vi "探头窗口-6-服务器版.vi"() -> ()   [LabVIEW 2013]
panel:
  in  "外部停止命令？":bool=TRUE
  out "引用-探头属性[]":refnum<vi>
  out "引用-监测模式？":refnum<vi>
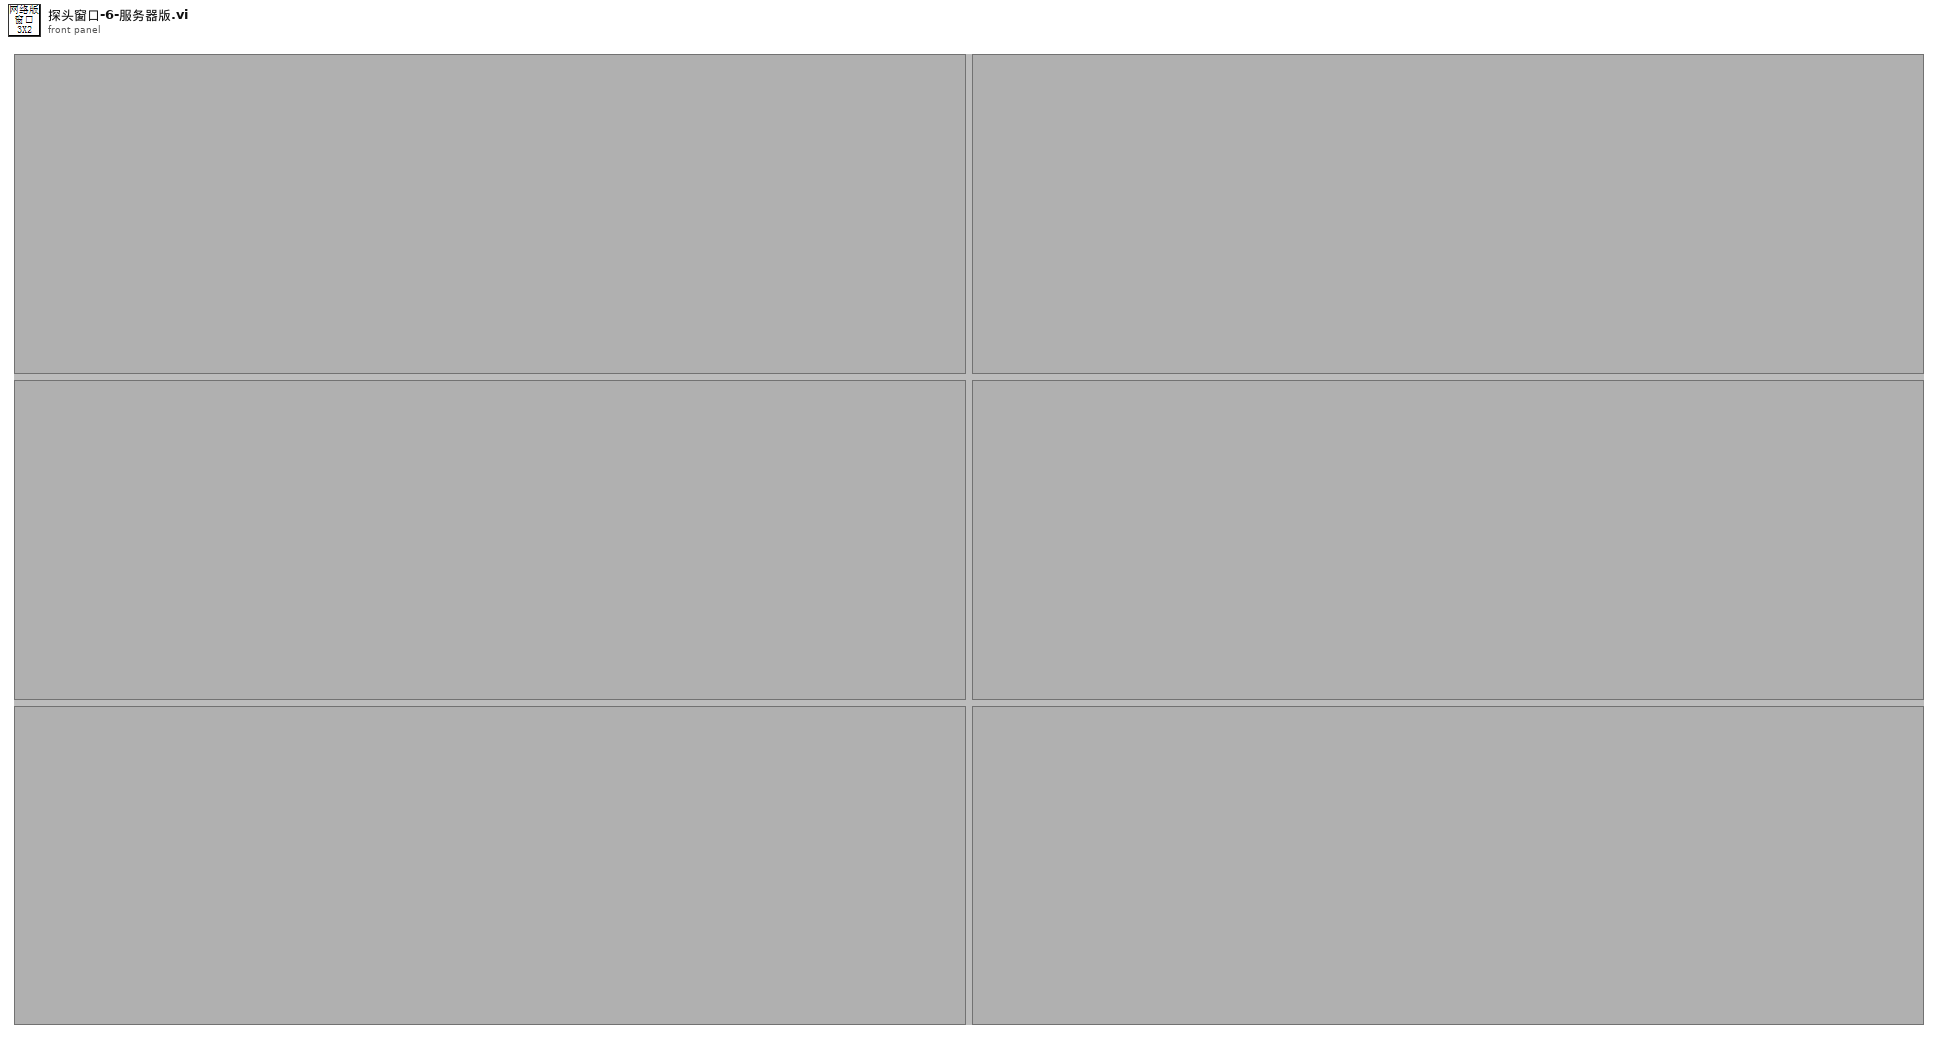
[diagram p1: front panel]
types:
  T1 = cluster{"探头地址与信息":cluster{"网络地址":cluster{"IP":string, "port":u16}, "探头信息":string}, "测量值":cluster{"时间":timestamp, "数值":dbl}, "限值":cluster{"限值1":dbl, "限值2":dbl}, "探头状态":enum16{"正常", "离线", "禁用", "一级报警", "二级报警"}}[]
  T2 = typedef "eventvkey.ctl" = enum16{"ASCII", "Enter", "Return", "Shift", "Ctrl", "Alt", "Cmd", "Opt", "Caps", "NumLock", "Clear", "Break", "Up", "Down", "Left", "Right", "Insert", "Delete", "Home", "End", "PageUp", "PageDown", "Escape", "Help", "Pause", "ScrollLock", "F1", "F2", "F3", "F4", "F5", "F6", "F7", "F8", "F9", "F10", "F11", "F12", "F13", "F14", "F15", "F16", "F17", "F18", "F19", "F20", "F21", "F22", "F23", "F24", "Play", "VolumeUp", "VolumeDown", "Mute", "Two Byte Char"}
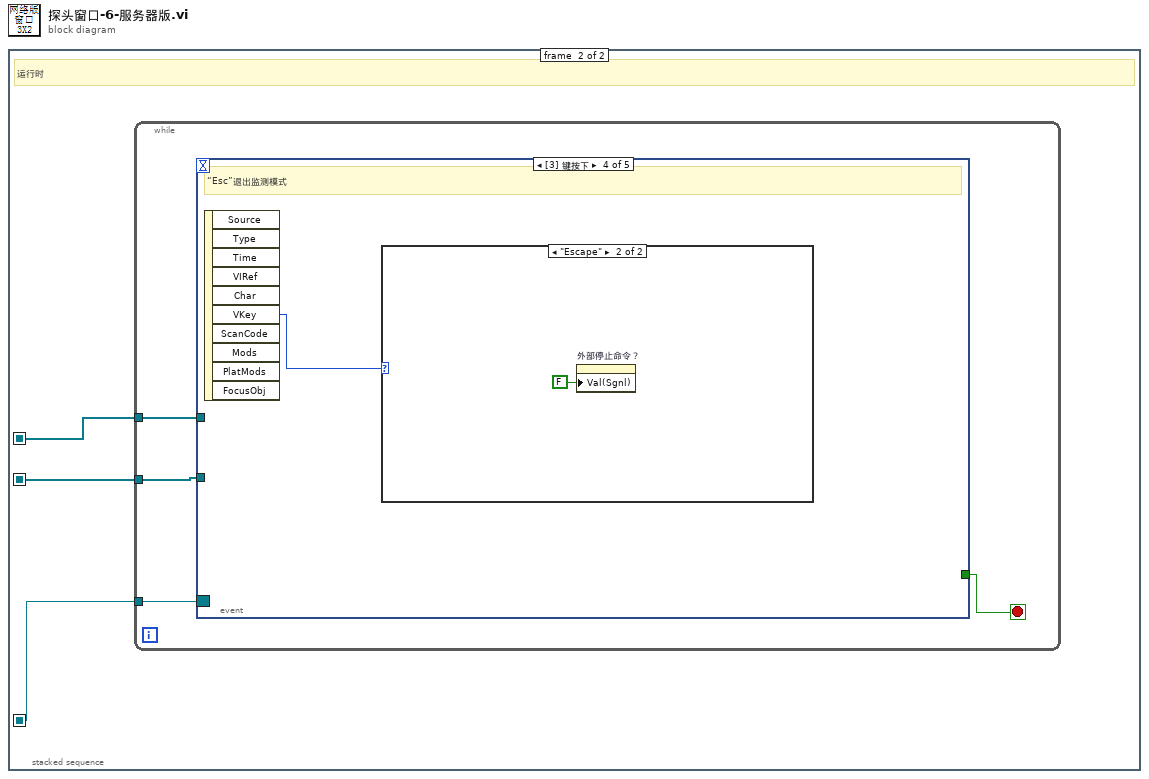
[diagram p0: block diagram]
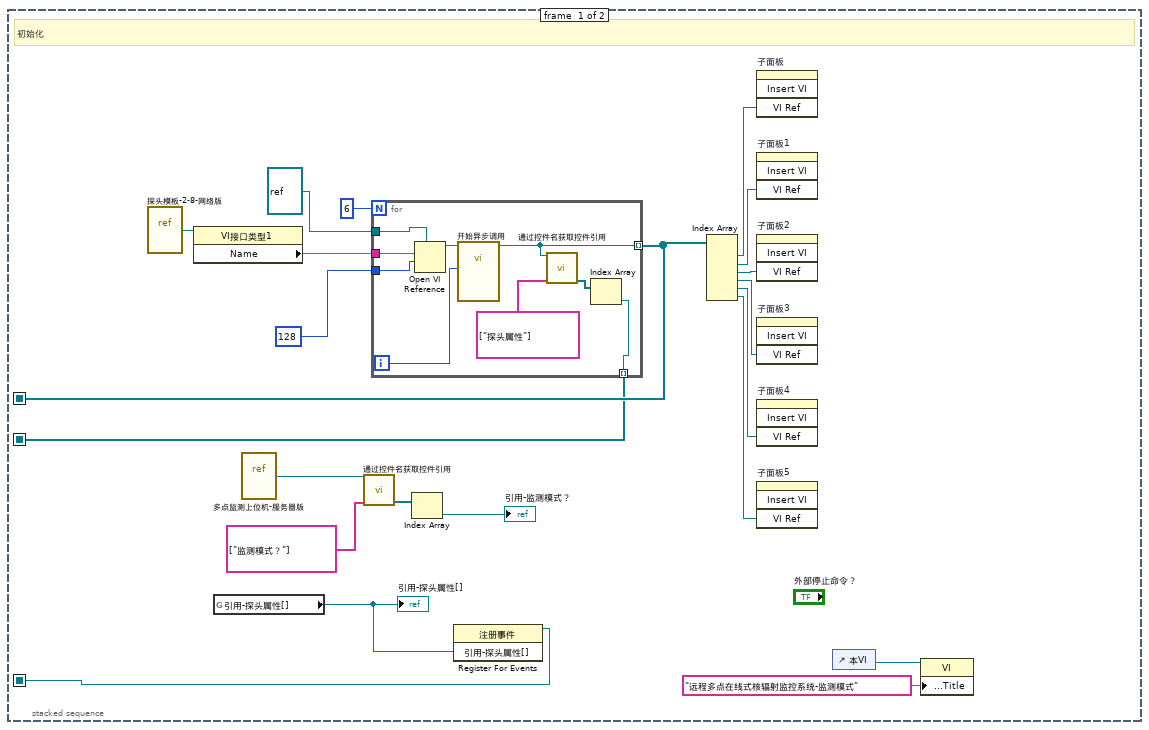
[diagram p2: hidden frame]
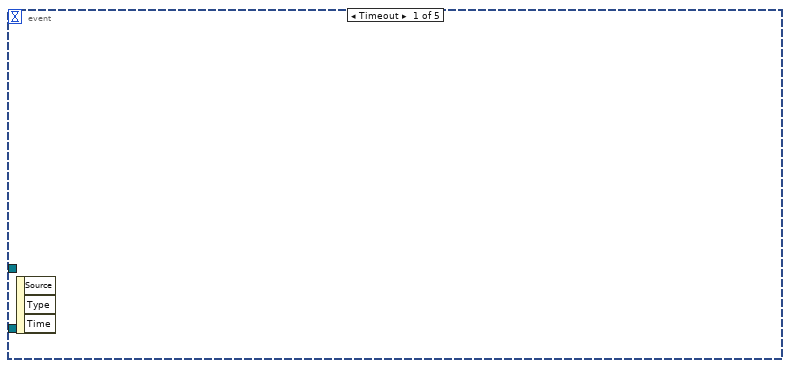
[diagram p3: hidden frame]
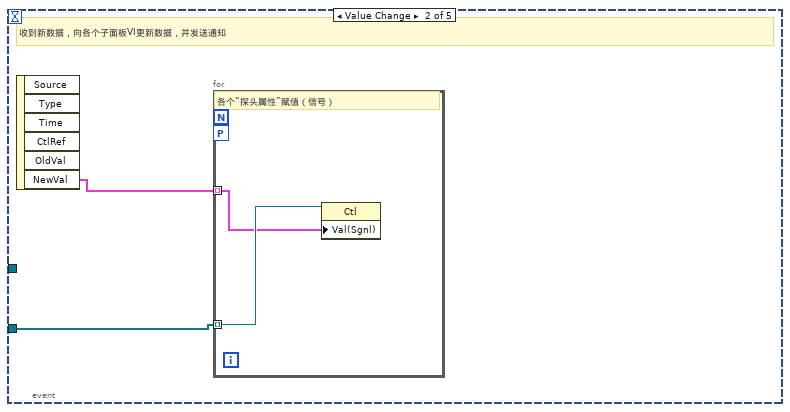
[diagram p4: hidden frame]
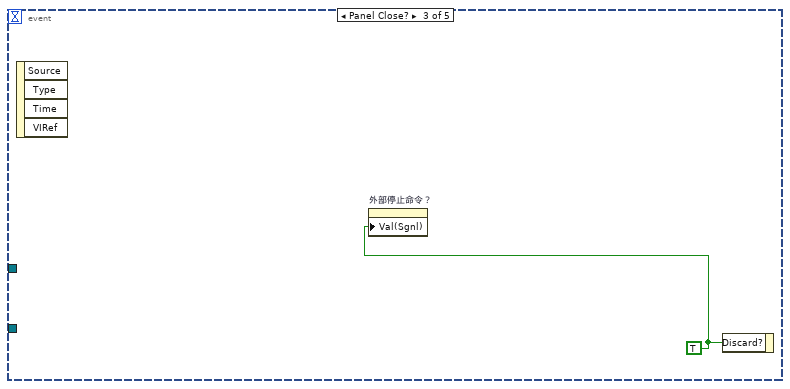
[diagram p5: hidden frame]
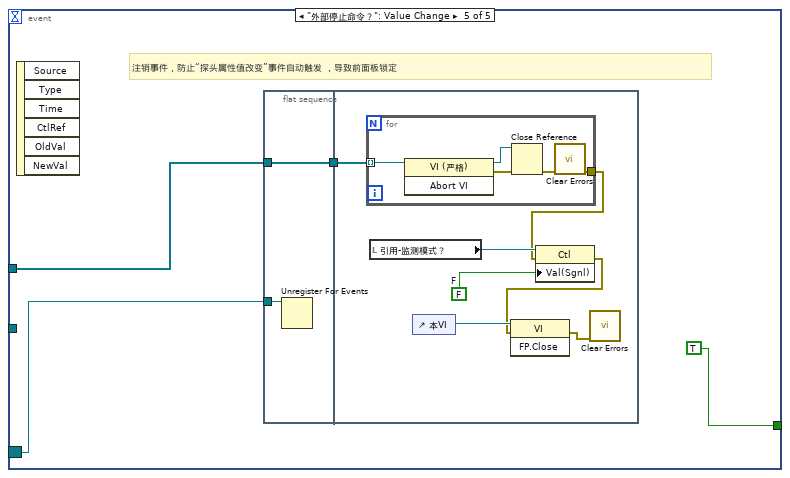
[diagram p7: hidden frame]
diagram:
  n1 = stacked-sequence {
    seq-local: [w17 _] -> [_ w33]
    seq-local: [w9 _] -> [_ w32]
    seq-local: [w3 _] -> [_ w31]
    frame #0 {
      # "初始化"
      n2 = vi-ref "探头模板-2-8-网络版.vi"() -> (w21:refnum<vi>)
      n3 = property class="VI接口类型1"(reference=w21) -> ("Name"=w20:string)  [unwired: 1 in, 2 out]
      n4 = global read "全局变量-35点监测.vi" "引用-探头属性[]"() -> (w4:refnum<vi>)
      "引用-探头属性[]" <- w4
      n5 = vi-ref "多点监测上位机-服务器版.vi"() -> (w5:refnum<vi>)
      n6 = call "通过控件名获取控件引用.vi"("控件名数组"=string[] ["监测模式？"], "VI引用"=w5) -> ("控件引用输出"=w7:refnum<vi>[])  [unwired: 7 in, 2 out]
      n7 = for {
        N: 6 -> [_]
        tunnel: w20 -> [w30]
        tunnel: 128 ("选项") -> [w29]
        tunnel: refnum<vi> refnum ("类型说明符VI引用句柄（仅用于类型）") -> [w28]
        tunnel: [w23] -> w17 mode=indexing
        tunnel: [w24] -> w9 mode=indexing
        i -> [w22]
        n8 = Open VI Reference(type specifier VI Refnum (for type only)=w28, vi path=w30, options=w29) -> (vi reference=w25:refnum<vi>)  [unwired: 3 in, 1 out]
        n9 = call-by-ref "开始异步调用"(reference=w25, "探头序号"=w22) -> (reference out=w23:refnum<vi>)  [unwired: 12 in, 1 out]
        n10 = call "通过控件名获取控件引用.vi"("控件名数组"=string[] ["探头属性"], "VI引用"=w23) -> ("控件引用输出"=w27:refnum<vi>[])  [unwired: 7 in, 2 out]
        n11 = Index Array(array=w27) -> (element=w24:refnum<vi>)  [unwired: 1 in]
      }
      n12 = Index Array(array=w7) -> (element=→"引用-监测模式？":refnum<vi>)  [unwired: 1 in]
      n13 = register-events(w4) -> (reference out=w3:refnum<event-registration>)  [unwired: 2 in, 1 out]
      n14 = Index Array(array=w17) -> (element #1=w15:refnum<vi>, element #2=w14:refnum<vi>, element #3=w13:refnum<vi>, element #4=w12:refnum<vi>, element #5=w10:refnum<vi>, element #6=w11:refnum<vi>)  [unwired: 6 in]
      n15 = invoke on="子面板" class="子面板" method="Insert VI"("VI Ref"=w15) -> ()  [unwired: 3 in, 4 out]
      n16 = invoke on="子面板1" class="SubPnl" method="Insert VI"("VI Ref"=w14) -> ()  [unwired: 3 in, 4 out]
      n17 = invoke on="子面板2" class="SubPnl" method="Insert VI"("VI Ref"=w13) -> ()  [unwired: 3 in, 4 out]
      n18 = invoke on="子面板3" class="SubPnl" method="Insert VI"("VI Ref"=w12) -> ()  [unwired: 3 in, 4 out]
      n19 = invoke on="子面板4" class="SubPnl" method="Insert VI"("VI Ref"=w10) -> ()  [unwired: 3 in, 4 out]
      n20 = invoke on="子面板5" class="SubPnl" method="Insert VI"("VI Ref"=w11) -> ()  [unwired: 3 in, 4 out]
      n21 = control-ref of="本VI"() -> (w2:refnum<vi>)
      n22 = property class="VI"(reference=w2, "Front Panel.Title"="远程多点在线式核辐射监控系统-监测模式" ("前面板窗口:标题")) -> ()  [unwired: 1 in, 2 out]
    }
    frame #1 {
      # "运行时"
      n23 = while {
        tunnel: w33 -> [w36]
        tunnel: w32 -> [w35]
        tunnel: w31 -> [w34]
        stop <- w37 stop-if-true
        n24 = event shown="[3] 键按下" {
          selector: w34 -> [_ _ _ _ w45]
          dyn-events: _ -> [_ _ _ _ _]
          timeout: _ -> [_ _ _ _ _]
          tunnel: [_ _ _ _ TRUE ("放弃？")] -> w37
          tunnel: w36 -> [_ _ _ _ w47]
          tunnel: w35 -> [_ w38 _ _ _]
          event Timeout {
            n25 = event-data() -> ()  [unwired: 1 in, 3 out]
          }
          event Value Change {
            # "收到新数据，向各个子面板VI更新数据，并发送通知"
            n26 = event-data() -> ("NewVal"=w39:T1)  [unwired: 1 in, 5 out]
            n27 = for {
              workers-P: _ -> [_]
              tunnel: w38 -> [w41] mode=indexing
              tunnel: w39 -> [w40] mode=indexing
              # "各个“探头属性”赋值（信号）"
              n28 = property class="Ctl"(reference=w41, "Val(Sgnl)"=w40) -> ()  [unwired: 1 in, 2 out]
            }
          }
          event Panel Close? {
            w42 = TRUE ("放弃？")
            n29 = event-data() -> ()  [unwired: 1 in, 4 out]
            n30 = property on="外部停止命令？" class="Bool (严格)"("Val(Sgnl)"=w42) -> ()  [unwired: 2 in, 2 out]
            n31 = event-data("Discard?"=w42) -> ()  [unwired: 1 in, 1 out]
          }
          event Key Down {
            # "“Esc”退出监测模式"
            n32 = event-data() -> ("VKey"=w43:T2)  [unwired: 1 in, 9 out]
            n33 = case shown="\"Escape\"" w43 {
              frame "ASCII", Default {
              }
              frame "Escape" {
                n34 = property on="外部停止命令？" class="Bool (严格)"("Val(Sgnl)"=FALSE ("值(信号)")) -> ()  [unwired: 2 in, 2 out]
              }
            }
          }
          event "外部停止命令？": Value Change {
            # "注销事件，防止“探头属性值改变”事件自动触发 ，导致前面板锁定"
            n35 = event-data() -> ()  [unwired: 1 in, 6 out]
            n36 = flat-sequence {
              tunnel: w47 -> [w50]
              tunnel: [w50] -> w46
              tunnel: w45 -> [w49]
              tunnel: w46 -> [w57]
              frame #0 {
                n37 = Unregister For Events(event registration refnum=w49) -> ()  [unwired: 1 in, 1 out]
              }
              frame #1 {
                w56 = FALSE  # F
                n38 = for {
                  tunnel: w57 -> [w62] mode=indexing
                  tunnel: [w58] -> w52
                  n39 = invoke class="VI (严格)" method="Abort VI"(reference=w62) -> (reference out=w60:refnum<vi>, error out=w61:errorcluster)  [unwired: 2 in, 1 out]
                  n40 = Close Reference(reference=w60, error in (no error)=w61) -> (error out=w59:errorcluster)
                  n41 = call <vilib>:"Clear Errors.vi"("error in (no error)"=w59) -> ("error out"=w58:errorcluster)  [unwired: 6 in]
                }
                n42 = local read "引用-监测模式？"() -> (w55:refnum<vi>)
                n43 = control-ref of="本VI"() -> (w54:refnum<vi>)
                n44 = property class="Ctl"(reference=w55, error in=w52, "Val(Sgnl)"=w56) -> (error out=w51:errorcluster)  [unwired: 1 out]
                n45 = invoke class="VI" method="FP.Close"(reference=w54, error in=w51) -> (error out=w53:errorcluster)  [unwired: 1 in, 2 out]
                n46 = call <vilib>:"Clear Errors.vi"("error in (no error)"=w53) -> ()  [unwired: 6 in, 1 out]
              }
            }
          }
        }
      }
    }
  }
